vi "CThread Activate FTC Functions.vi"(11 "NXT":T1={"Hardware"="NXT", "Flattened String"=""}) -> (3 "NXT":T1={"Hardware"="NXT", "Flattened String"=""})   [LabVIEW 2010, in "FTC.lvlib"]
uses:
  FTC.lvlib
  <vilib>/NXT/Subs/LVHSConnector.ctl
  CLIB/CThread/Core/CThread Thread Properties.ctl
  CLIB/CRef/Interface/CRef Boolean.llb/Boolean CReference.ctl
  CLIB/CThread/XNodes/referencenode/CThread VI Reference.xnode
  CLIB/CThread/XNodes/terminalnode/CThread VI Terminal Node.xnode
  CLIB/CThread/Base/CThread Base - VI Reference.vi
  CLIB/CThread/Base/CThread Base - While Loop.vi
  CLIB/CThread/CThread.lvlib
  CLIB/CRef/CRef.lvlib
  CLIB/CRef/Interface/CRef Numeric.llb/I32 CReference.ctl
  Process All FTC Functions.vi
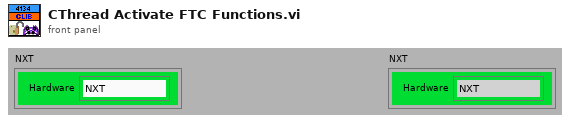
[diagram p1: front panel]
types:
  T1 = typedef "LVHSConnector.ctl" = cluster{"Hardware":string, "Flattened String":string}
  T2 = typedef "CThread.lvlib/CThread Thread Properties.ctl" = cluster{"Post-Run Delay (5ms)":u32}
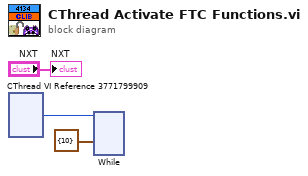
[diagram p0: block diagram]
diagram:
  n1 = xnode "CThread VI Reference 3771799909"() -> ("..\\Process All FTC Functions.vi"=w1:i32)
  n2 = xnode "While"("CLIB VI Reference"=w1, "Thread Properties"=T2 {"Post-Run Delay (5ms)"=10}) -> ()  [unwired: 1 in, 2 out]
  "NXT" <- "NXT"
